vi "Compact Logging.vi"(8 "error in":errorcluster, 11 "DIG_IO in":refnum<class "DIG_IO.lvclass">) -> (0 "error out":errorcluster, 2 "Compact Record":waveform(i16)[](array[waveform]), 3 "DIG_IO out":refnum<class "DIG_IO.lvclass">)   [LabVIEW 2019, in "DIG_IO.lvlib" / "DIG_IO.lvclass"]
uses:
  Library/DIG_IO.lvclass
  C:/Users/Public/Documents/Development/builds/Instruments/Instruments.lvlibp/Library/Instruments.lvclass
  Library/DIG_IO.lvclass/DIG_IO.ctl
  Accessors/Read Banks.vi
  builds/Instruments/Instruments.lvlibp/Accessors/Read dt.vi
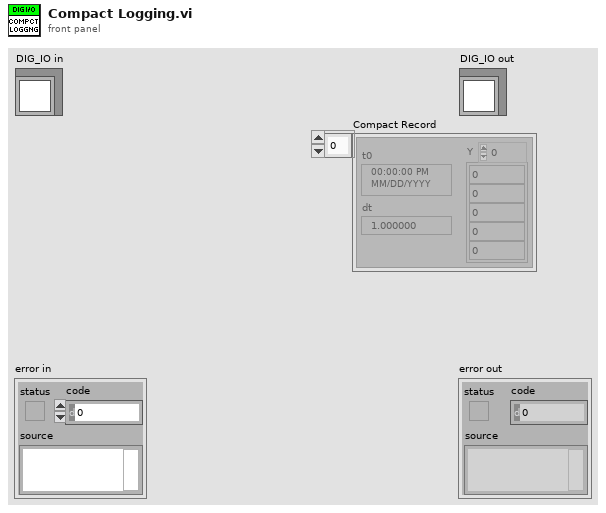
[diagram p1: front panel]
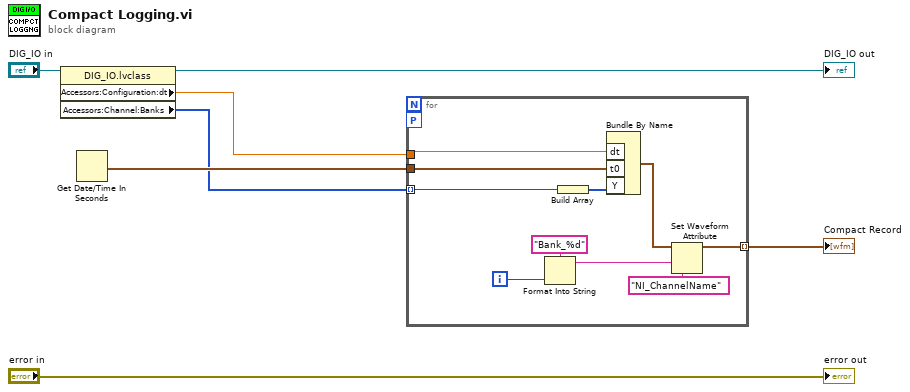
[diagram p0: block diagram]
diagram:
  n1 = property class="DIG_IO.lvclass"(reference="DIG_IO in") -> (reference out=→"DIG_IO out":refnum<class "DIG_IO.lvclass">, "Accessors:Configuration:dt"=w6:dbl, "Accessors:Channel:Banks"=w1:u8[])  [unwired: 1 in, 1 out]
  n2 = Get Date/Time In Seconds() -> (seconds since 1Jan1904=w7:timestamp)
  n3 = for {
    tunnel: w1 -> [w17] mode=indexing
    tunnel: [w15] -> w2 mode=indexing
    tunnel: w7 -> [w11]
    workers-P: _ -> [_]
    tunnel: w6 -> [w13]
    i -> [w9]
    n4 = Format Into String(format string="Bank_%d", w9) -> (resulting string=w8:string)  [unwired: 2 in, 1 out]
    n5 = Build Array(w17) -> (w12:u8[])
    n6 = Bundle By Name("dt"=w13, "t0"=w11, "Y"=w12) -> (w16:waveform(u8))  [unwired: 1 in]
    n7 = Set Waveform Attribute(5:w8, 6:"NI_ChannelName" ("name"), 7:w16) -> (3:w15:waveform(u8))  [unwired: 1 in, 2 out]
  }
  "Compact Record" <- w2
  "error out" <- "error in"
